vi "Helper - AngleInRange.vi"(9 "Angle to check":dbl, 10 "Angle 2":dbl, 11 "Angle 1":dbl) -> (2 "In range?":bool)   [LabVIEW 2011]
doc: "Takes in wind angle + irons range and wind angle - irons range, both normalized to be within 0-360, and checks whether the angle inputed falls within the irons range."
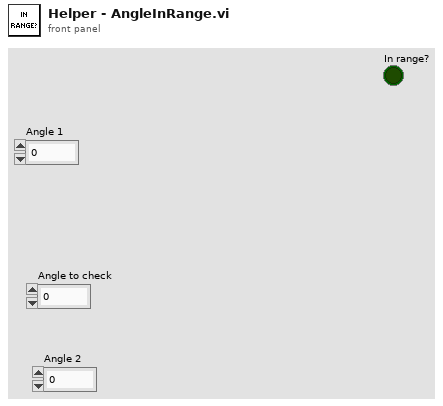
[diagram p1: front panel]
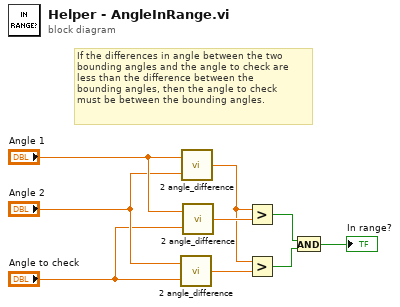
[diagram p0: block diagram]
diagram:
  # "If the differences in angle between the two\nbounding angles and the angle to check are \nless than the difference between the\nbounding angles, then the angle to check\nmust be between the bounding angles."
  n1 = call "2 angle_difference.vi"("Angle 2"="Angle to check", "Angle 1"="Angle 2") -> ("Difference"=w5:dbl)
  n2 = call "2 angle_difference.vi"("Angle 2"="Angle 2", "Angle 1"="Angle 1") -> ("Difference"=w4:dbl)
  n3 = call "2 angle_difference.vi"("Angle 2"="Angle to check", "Angle 1"="Angle 1") -> ("Difference"=w6:dbl)
  n4 = Greater?(x=w4, y=w6) -> (0:w2:bool)
  n5 = Greater?(x=w4, y=w5) -> (0:w3:bool)
  n6 = And(x=w2, y=w3) -> (x .and. y?=→"In range?":bool)
